vi "GenerateTimeAndDateCSV_LDO.vi"(8 "error in (no error)":errorcluster, 11 "Test string input":string) -> (0 "error out":errorcluster, 3 "path for csv file":path)   [LabVIEW 2023, in "WritingDataFile.lvlib"]
uses:
  WritingDataFile.lvlib
  <vilib>/Utility/error.llb/whitespace.ctl
  <vilib>/Utility/error.llb/Trim Whitespace One-Sided.vi
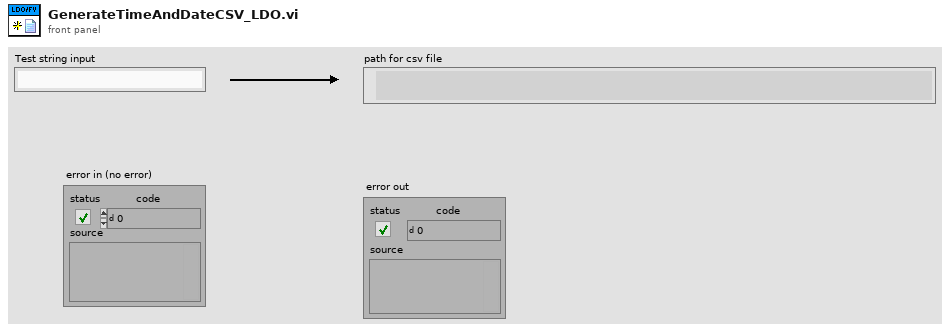
[diagram p1: front panel]
types:
  T1 = typedef "whitespace.ctl" = u16
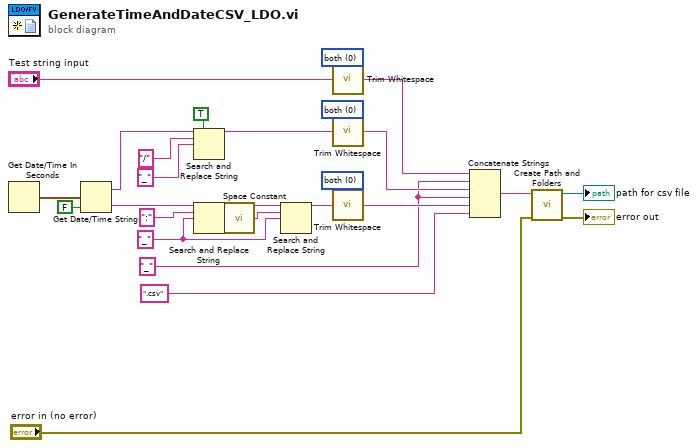
[diagram p0: block diagram]
diagram:
  w8 = T1 0 items=["both", "start of string", "end of string"] ("location (both)")
  w11 = T1 0 items=["both", "start of string", "end of string"] ("location (both)")
  w13 = T1 0 items=["both", "start of string", "end of string"] ("location (both)")
  w14 = "_" ("replace string (\"\")")
  w4 = "_"
  n1 = Get Date/Time In Seconds() -> (seconds since 1Jan1904=w24:timestamp)
  n2 = Get Date/Time String(seconds (now)=w24, want seconds? (F)=FALSE) -> (date string=w21:string, time string=w26:string)  [unwired: 1 in]
  n3 = Search and Replace String(replace all?=TRUE ("replace all? (F)"), input string=w21, search string="/", replace string="_" ("replace string (\"\")")) -> (result string=w10:string)  [unwired: 4 in, 3 out]
  n4 = Search and Replace String(input string=w26, search string=":", replace string=w14) -> (result string=w16:string)  [unwired: 5 in, 3 out]
  n5 = call <vilib>:"Space Constant.vi"() -> ("String"=w15:string)
  n6 = Search and Replace String(input string=w16, search string=w15, replace string=w14) -> (result string=w7:string)  [unwired: 5 in, 3 out]
  n7 = call <vilib>:"Trim Whitespace.vi"("string"="Test string input", "location (both)"=w13) -> ("trimmed string"=w12:string)
  n8 = call <vilib>:"Trim Whitespace.vi"("string"=w10, "location (both)"=w11) -> ("trimmed string"=w9:string)
  n9 = call <vilib>:"Trim Whitespace.vi"("string"=w7, "location (both)"=w8) -> ("trimmed string"=w6:string)
  n10 = Concatenate Strings(w12, w4, w9, w4, w6, ".csv" ("string")) -> (w5:string)
  n11 = call "Create Path and Folders.vi"("error in (no error)"="error in (no error)", "String Path"=w5) -> ("error out"=→"error out":errorcluster, "path for csv file"=→"path for csv file":path)  [unwired: 8 in]
